vi "Set Server Address.vi"(10 "Server Address":string, 11 "OOP Server in":refnum<class "OCVServer.lvclass">) -> (3 "OOP Server out":refnum<class "OCVServer.lvclass">)   [LabVIEW 2019, in "OCVServer.lvlib" / "OCVServer.lvclass"]
uses:
  OCVServer.lvclass
  OCVServer.lvclass/OCVServer.ctl
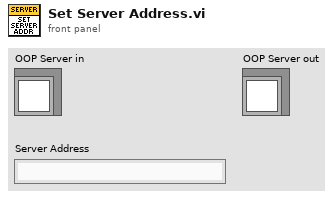
[diagram p1: front panel]
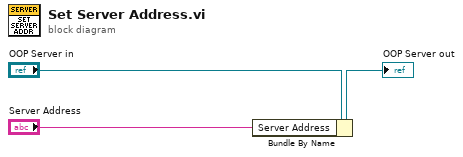
[diagram p0: block diagram]
diagram:
  n1 = Bundle By Name(cluster="OOP Server in", "Server Address"="Server Address") -> (→"OOP Server out":refnum<class "OCVServer.lvclass">)
